vi "Cluster_Array-1D_Array.vi"(8 "Plotter Selector":u16(ring) items=["High Voltage", "High Voltage PS", "Chain Current", "Column Current", "Lost Charge", "Radiation", "Pressure", "HV Control Difference"], 11 "Input Cluster":T1(array[cluster])) -> (0 "Output Data":dbl[](array[numeric]), 1 "Time":dbl[](array[numeric]))   [LabVIEW 2012, in "AccelNET.lvlib" / "Useful_SubVIs.lvlib"]
uses:
  Useful_SubVIs.lvlib
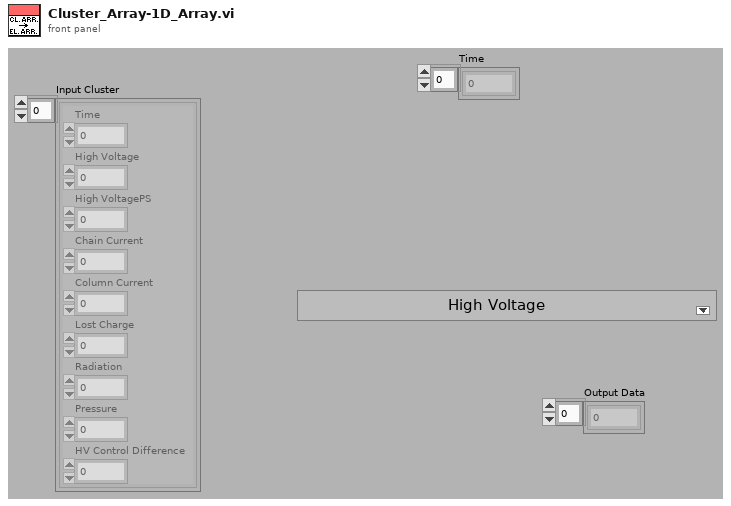
[diagram p1: front panel]
types:
  T1 = cluster{"Time":dbl, "High Voltage":dbl, "High VoltagePS":dbl, "Chain Current":dbl, "Column Current":dbl, "Lost Charge":dbl, "Radiation":dbl, "Pressure":dbl, "HV Control Difference":dbl}[]
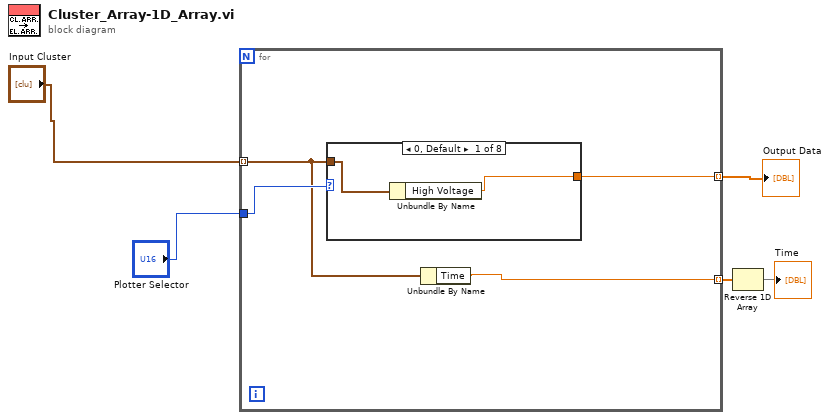
[diagram p0: block diagram]
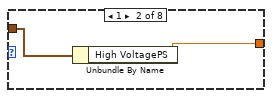
[diagram p2: hidden frame]
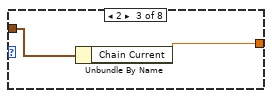
[diagram p3: hidden frame]
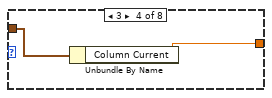
[diagram p4: hidden frame]
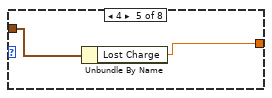
[diagram p5: hidden frame]
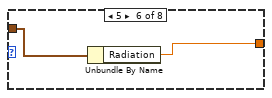
[diagram p6: hidden frame]
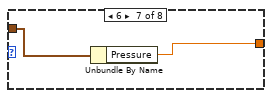
[diagram p7: hidden frame]
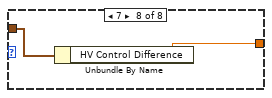
[diagram p8: hidden frame]
diagram:
  n1 = for {
    tunnel: "Input Cluster" -> [w7] mode=indexing
    tunnel: "Plotter Selector" -> [w9]
    tunnel: [w8] -> w4 mode=indexing
    tunnel: [w6] -> w2 mode=indexing
    n2 = case shown="0, Default" w9 {
      tunnel: w7 -> [w11 w13 w15 w17 w19 w21 w23 w25]
      tunnel: [w10 w12 w14 w16 w18 w20 w22 w24] -> w8
      frame 0, Default {
        n3 = Unbundle By Name(w11) -> ("High Voltage"=w10:dbl)
      }
      frame 1 {
        n4 = Unbundle By Name(w13) -> ("High VoltagePS"=w12:dbl)
      }
      frame 2 {
        n5 = Unbundle By Name(w15) -> ("Chain Current"=w14:dbl)
      }
      frame 3 {
        n6 = Unbundle By Name(w17) -> ("Column Current"=w16:dbl)
      }
      frame 4 {
        n7 = Unbundle By Name(w19) -> ("Lost Charge"=w18:dbl)
      }
      frame 5 {
        n8 = Unbundle By Name(w21) -> ("Radiation"=w20:dbl)
      }
      frame 6 {
        n9 = Unbundle By Name(w23) -> ("Pressure"=w22:dbl)
      }
      frame 7 {
        n10 = Unbundle By Name(w25) -> ("HV Control Difference"=w24:dbl)
      }
    }
    n11 = Unbundle By Name(w7) -> ("Time"=w6:dbl)
  }
  "Output Data" <- w4
  n12 = Reverse 1D Array(array=w2) -> (reversed array=→"Time":dbl[])
